vi "GDSString_EnumsToStringsValue.vi"(0 "VariantIn(Enum(s) or String(s), could be an array)":variant, 5 "error in (no error)":errorcluster) -> (14 "StringOut":string, 15 "StringsOut":string[](array[string]), 19 "error out":errorcluster)   [LabVIEW 2020]
doc: "Uses a flatten XML string of a Enum-type <B>\"XmlEnumStringIn\"</B> to find the acctually value of the enum.\nThis is normally used when a Enum has been flatten to a variant.\nIt could also take the enum variant as an input\nIt the Variant ENUM is of string type it will send it through without any errors"
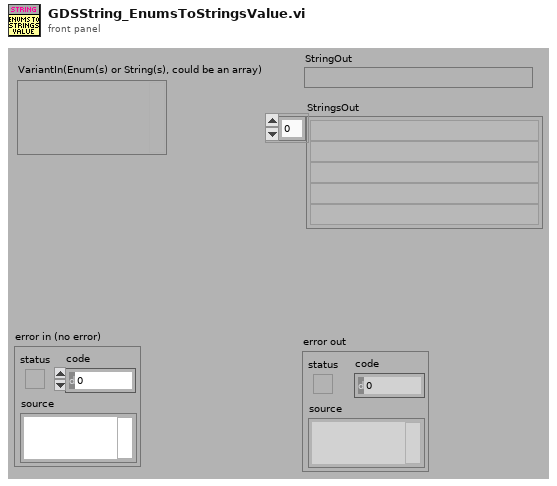
[diagram p1: front panel]
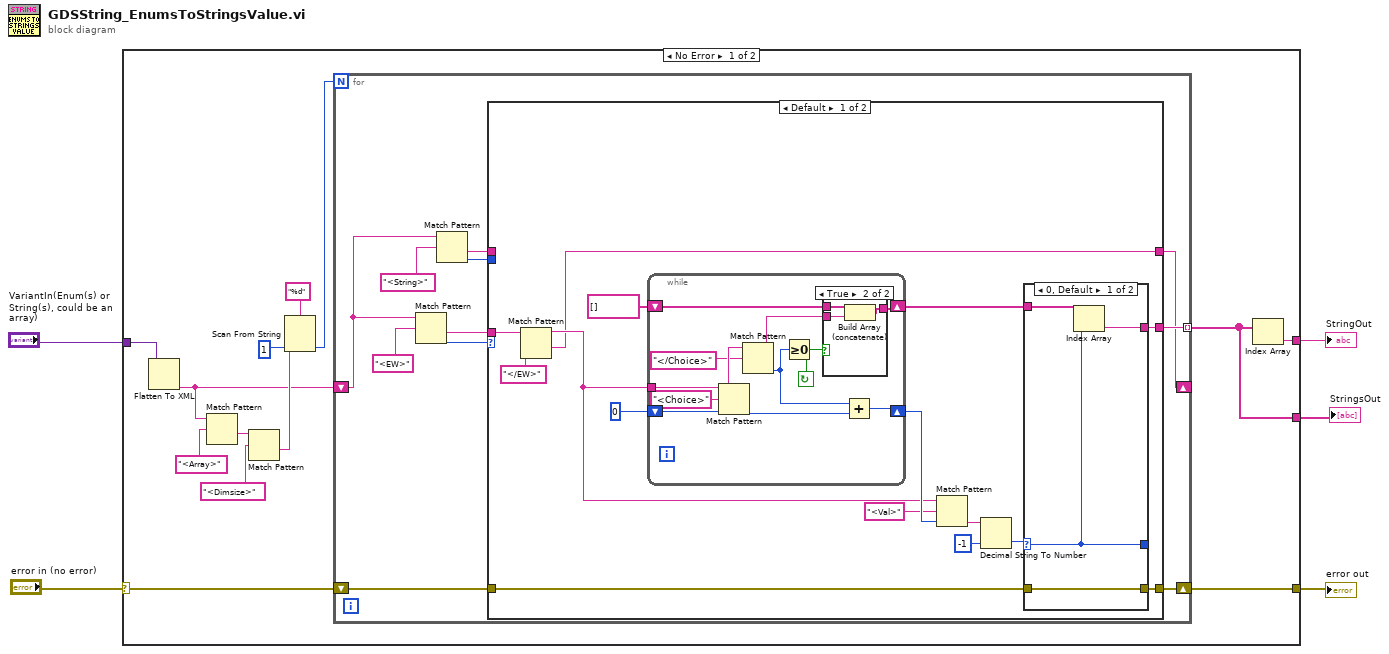
[diagram p0: block diagram]
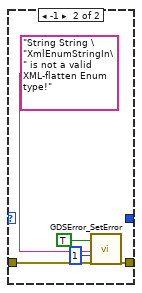
[diagram p2: hidden frame]
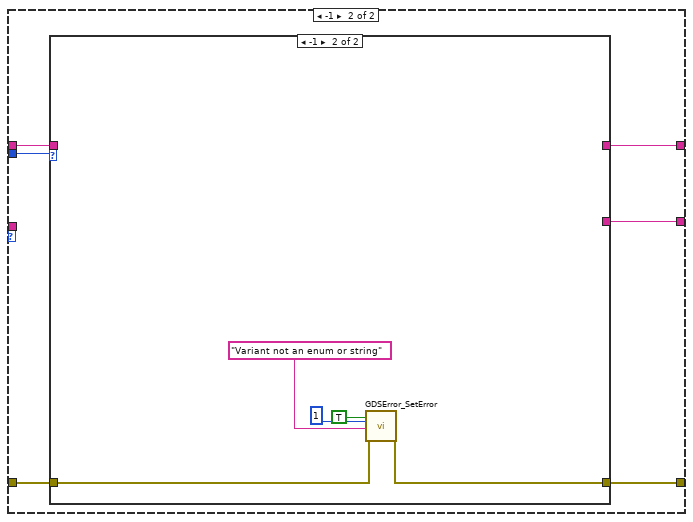
[diagram p4: hidden frame]
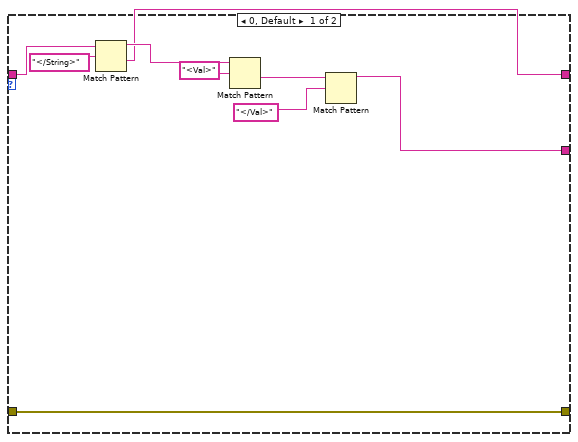
[diagram p5: hidden frame]
diagram:
  n1 = case shown="No Error" "error in (no error)" {
    selector: "error in (no error)" -> [w11 w90]
    tunnel: [w12 w90] -> w4
    tunnel: [w15 _] -> w3
    tunnel: "VariantIn(Enum(s) or String(s), could be an array)" -> [w18 _]
    tunnel: [w16 _] -> w1
    frame No Error {
      n2 = Flatten To XML(6:w18) -> (2:w6:string)
      n3 = Match Pattern(string=w6, regular expression="<Array>") -> (after substring=w14:string)  [unwired: 1 in, 3 out]
      n4 = Match Pattern(string=w14, regular expression="<Dimsize>") -> (after substring=w10:string)  [unwired: 1 in, 3 out]
      n5 = Scan From String(format string="%d", input string=w10, default 1=1) -> (output 1=w8:i32)  [unwired: 2 in, 3 out]
      n6 = for {
        N: w8 -> [_]
        tunnel: [w27] -> w16 mode=indexing
        shift-right: [w24] -> w12
        shift-left: w11 -> [w23]
        shift-right: [w20] -> _
        shift-left: w6 -> [w21]
        n7 = Match Pattern(string=w21, regular expression="<EW>") -> (after substring=w22:string, offset past match=w28:i32)  [unwired: 1 in, 2 out]
        n8 = Match Pattern(string=w21, regular expression="<String>") -> (after substring=w19:string, offset past match=w25:i32)  [unwired: 1 in, 2 out]
        n9 = case shown="Default" w28 {
          tunnel: w23 -> [w37 w75]
          tunnel: [w36 w74] -> w24
          tunnel: [w35 w72] -> w27
          tunnel: w25 -> [_ w73]
          tunnel: w22 -> [w33 _]
          tunnel: [w30 w70] -> w20
          tunnel: w19 -> [_ w71]
          frame Default {
            n10 = Match Pattern(string=w33, regular expression="</EW>") -> (before substring=w31:string, after substring=w30:string)  [unwired: 1 in, 2 out]
            n11 = while {
              shift-left: 0 ("offset past match") -> [w63]
              shift-right: [w59] -> w42
              tunnel: w31 -> [w64]
              shift-right: [w55] -> w34
              shift-left: string[] [] -> [w56]
              stop <- w57 continue-if-true
              n12 = Match Pattern(string=w64, regular expression="<Choice>", offset (0)=w63) -> (after substring=w62:string, offset past match=w60:i32)  [unwired: 2 out]
              n13 = Match Pattern(string=w62, regular expression="</Choice>") -> (before substring=w54:string, offset past match=w58:i32)  [unwired: 1 in, 2 out]
              n14 = Greater Or Equal To 0?(x=w58) -> (x >= 0?=w57:bool)
              n15 = case shown="True" w57 {
                tunnel: w56 -> [w66 w69]
                tunnel: [w66 w68] -> w55
                tunnel: w54 -> [_ w67]
                frame False {
                }
                frame True {
                  n16 = Build Array (concatenate)(w69, w67) -> (w68:string[])
                }
              }
              n17 = Add(x=w58, y=w60) -> (x+y=w59:i32)
            }
            n18 = Match Pattern(string=w31, regular expression="<Val>", offset (0)=w42) -> (after substring=w40:string)  [unwired: 3 out]
            n19 = Decimal String To Number(string=w40, default (0L)=-1 ("default (0 I32)")) -> (number=w38:i32)  [unwired: 1 in, 1 out]
            n20 = case shown="0, Default" w38 {
              selector: w38 -> [w45 _]
              tunnel: w37 -> [w48 w50]
              tunnel: [w48 w49] -> w36
              tunnel: w34 -> [w47 _]
              tunnel: [w46 _] -> w35
              tunnel: [w45 _] -> _
              frame 0, Default {
                n21 = Index Array(array=w47, index=w45) -> (element=w46:string)
              }
              frame -1 {
                n22 = call <resource>:"GDSError_SetError.vi"("status"=TRUE, "code (5000)"=1, "source"="String String \"XmlEnumStringIn\" is not a valid XML-flatten Enum type!", "error in (no error)"=w50) -> ("error out"=w49:errorcluster)  [unwired: 15 in]
              }
            }
          }
          frame -1 {
            n23 = case shown="-1" w73 {
              tunnel: w75 -> [w80 w89]
              tunnel: [w80 w88] -> w74
              tunnel: [w81 _] -> w72
              tunnel: w71 -> [w79 _]
              tunnel: [w76 _] -> w70
              frame 0, Default {
                n24 = Match Pattern(string=w79, regular expression="</String>") -> (before substring=w77:string, after substring=w76:string)  [unwired: 1 in, 2 out]
                n25 = Match Pattern(string=w77, regular expression="<Val>") -> (after substring=w83:string)  [unwired: 1 in, 3 out]
                n26 = Match Pattern(string=w83, regular expression="</Val>") -> (before substring=w81:string)  [unwired: 1 in, 3 out]
              }
              frame -1 {
                n27 = call <resource>:"GDSError_SetError.vi"("status"=TRUE, "code (5000)"=1, "source"="Variant not an enum or string", "error in (no error)"=w89) -> ("error out"=w88:errorcluster)  [unwired: 15 in]
              }
            }
          }
        }
      }
      n28 = Index Array(array=w16) -> (element=w15:string)  [unwired: 1 in]
    }
    frame Error {
    }
  }
  "error out" <- w4
  "StringOut" <- w3
  "StringsOut" <- w1
